vi "Cross Power.vi"   [LabVIEW 2017, in "NI_AALPro.lvlib"]
doc: "Computes the cross power spectrum, <B>Sxy</B>, of the input signals <B>X</B> and <B>Y</B>. Wire data to the <B>X</B> input to determine the polymorphic instance to use or manually select the instance."
uses:
  NI_AALPro.lvlib
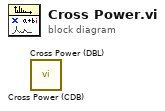
[diagram p0: block diagram]
diagram:
  n1 = call "Cross Power (CDB).vi"() -> ()  [unwired: 2 in, 2 out]
  n2 = call "Cross Power (DBL).vi"() -> ()  [unwired: 2 in, 2 out]
